vi "Cal_curve.vi"(11 "Formula of Calibration Curve":string) -> (3 "Raman freq (cm-1)":dbl)   [LabVIEW 2012]
uses:
  variables/GlobalUI.vi
  <vilib>/gmath/NI_Gmath.lvlib
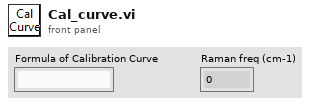
[diagram p1: front panel]
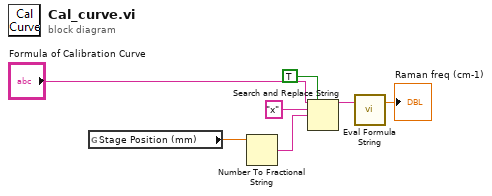
[diagram p0: block diagram]
diagram:
  n1 = global read "GlobalUI.vi" "Stage Position (mm)"() -> (w3:dbl)
  n2 = Number To Fractional String(number=w3) -> (F-format string=w5:string)  [unwired: 3 in]
  n3 = Search and Replace String(replace all?=TRUE ("replace all? (F)"), input string="Formula of Calibration Curve", search string="x", replace string=w5) -> (result string=w4:string)  [unwired: 4 in, 3 out]
  n4 = call <vilib>:"Eval Formula String.vi"("formula"=w4) -> ("y value"=→"Raman freq (cm-1)":dbl)  [unwired: 1 in, 1 out]
